vi "ConfirmShutdown.vi"(1 "Boolean":bool) -> (0 "OK Button 2":bool)   [LabVIEW 2025]
panel:
  in  "Cancel Button":bool
  in  "OK Button":bool
  # "Are you shure you want to shut down?"
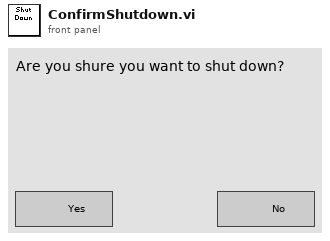
[diagram p1: front panel]
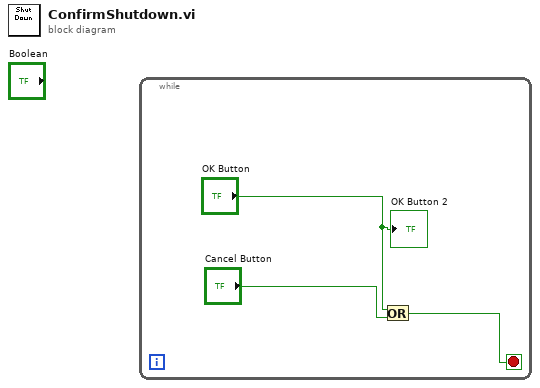
[diagram p0: block diagram]
diagram:
  n1 = while {
    stop <- w2 stop-if-true
    n2 = Or(x="OK Button", y="Cancel Button") -> (x .or. y?=w2:bool)
    "OK Button 2" <- "OK Button"
  }
